vi "Write State.vi"(10 "state:":T1, 11 "Model in":refnum<class "Model.lvclass">) -> (3 "Model out":refnum<class "Model.lvclass">)   [LabVIEW 2015, in "Model.lvclass"]
uses:
  Model.lvclass
  Typedefs/StateSelector.ctl
  Model.lvclass/Model.ctl
  Typedefs/FAMTTypedefs.lvlib
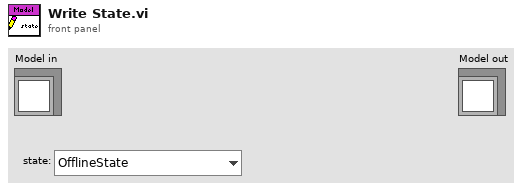
[diagram p1: front panel]
types:
  T1 = typedef "FAMTTypedefs.lvlib/StateSelector.ctl" = enum16{"OfflineState", "FaultState", "StandbyState", "DisabledState", "EnabledState", "WaitForUserInputState", "PerformOpenLoopScanState"}
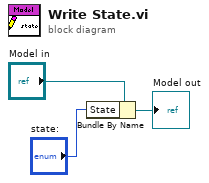
[diagram p0: block diagram]
diagram:
  n1 = Bundle By Name(cluster="Model in", "State"="state:") -> (→"Model out":refnum<class "Model.lvclass">)
